vi "PipBoy_DefaultValuesFileConf.vi"(8 "error in (no error)":errorcluster) -> (0 "error out":errorcluster, 2 "FileConf":T1)   [LabVIEW 2014]
uses:
  ctls/PipBoy_FileConf.ctl
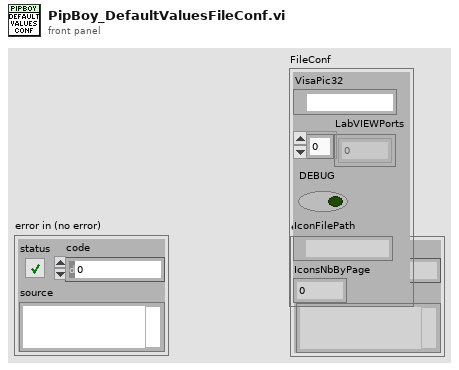
[diagram p1: front panel]
types:
  T1 = typedef "PipBoy_FileConf.ctl" = cluster{"VisaPic32":refnum<visa-resource-name>, "LabVIEWPorts":u16[], "DEBUG":bool, "IconFilePath":path, "IconsNbByPage":i32}
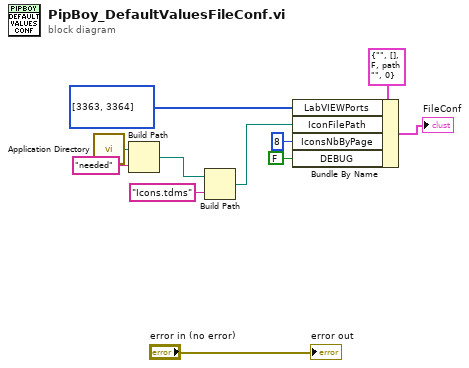
[diagram p0: block diagram]
diagram:
  n1 = call <vilib>:"Application Directory.vi"() -> ("Application Directory"=w7:path)
  n2 = Build Path(base path=w7, name or relative path="needed") -> (appended path=w5:path)
  n3 = Build Path(base path=w5, name or relative path="Icons.tdms") -> (appended path=w3:path)
  n4 = Bundle By Name(cluster=T1 {"VisaPic32"="", "LabVIEWPorts"=[], "DEBUG"=FALSE, "IconFilePath"=path "", "IconsNbByPage"=0} ("FileConf"), "LabVIEWPorts"=u16[] [3363, 3364], "IconFilePath"=w3, "IconsNbByPage"=8, "DEBUG"=FALSE) -> (→"FileConf":T1)
  "error out" <- "error in (no error)"
